vi "IsValidFolder.vi"(8 "error in (no error)":errorcluster, 11 "Source Path":path) -> (0 "error out":errorcluster, 2 "Valid Folder":bool, 3 "path out":path)   [LabVIEW 2023]
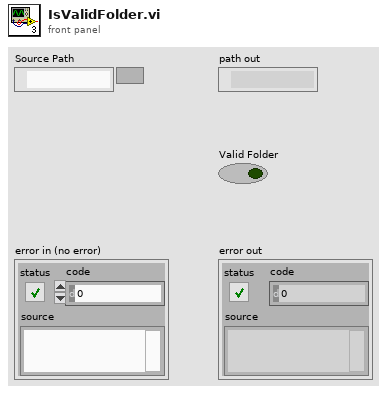
[diagram p1: front panel]
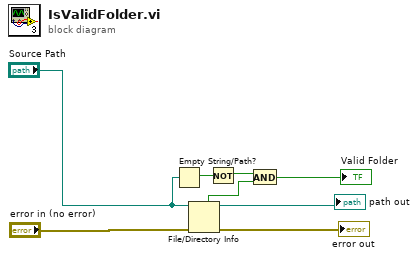
[diagram p0: block diagram]
diagram:
  n1 = Empty String/Path?(string/path="Source Path") -> (empty?=w3:bool)
  n2 = File/Directory Info(path="Source Path", error in="error in (no error)") -> (path out=→"path out":path, directory=w5:bool, error out=→"error out":errorcluster)  [unwired: 4 out]
  n3 = Not(x=w3) -> (.not. x?=w4:bool)
  n4 = And(x=w4, y=w5) -> (x .and. y?=→"Valid Folder":bool)
